vi "示波器2 - 副本 - 副本.vi"() -> ()   [LabVIEW 2018]
uses:
  <instrlib>/niScope/Configure/Trigger/niScope Configure Trigger Edge.vi
  <instrlib>/niScope/Acquire/niScope Multi Read WDT.vi
panel:
  in  "Channel(s) 2":string="0" caption="触发通道"
  out "Waveform From Scope 3":waveform(dbl)(graph) caption="采集通道"
  out "Waveform From Scope 2":waveform(dbl)(graph) caption="触发"
  out "error out":errorcluster
  in  "Channel(s)":string="0" caption="采集通道"
  out "Waveform From Scope":waveform(dbl)[](graph) caption="采集通道"
  in  "Vertical Range (V)":dbl=5.0 format="%_3g"
  in  "Min. Sample Rate":dbl=10000000.0 format="%#_6p"
  in  "Min Record Length":i32=40000
  in  "Vertical Coupling":i32(ring)=1 items=["AC", "DC", "Ground"]
  in  "Trigger Slope":i32(ring) items=["Positive", "Negative"]
  in  "Coupling":u16(ring)=1 items=["AC"=0, "DC"=1, "HF Reject"=3, "LF Reject"=4, "AC Plus HF Reject"=1001]
  in  "Trigger Level (V)":dbl=0.5 caption="Trigger Level" format="%.2f"
  in  "Trigger Modifier":i32(ring)=2 items=["None"=1, "Auto Trigger"=2]
  in  "Input Impedance":u32(ring) items=["1 mega ohm"=0, "50 ohms"=2]
  in  "Resource Name":refnum<k15>="DAQ::1"
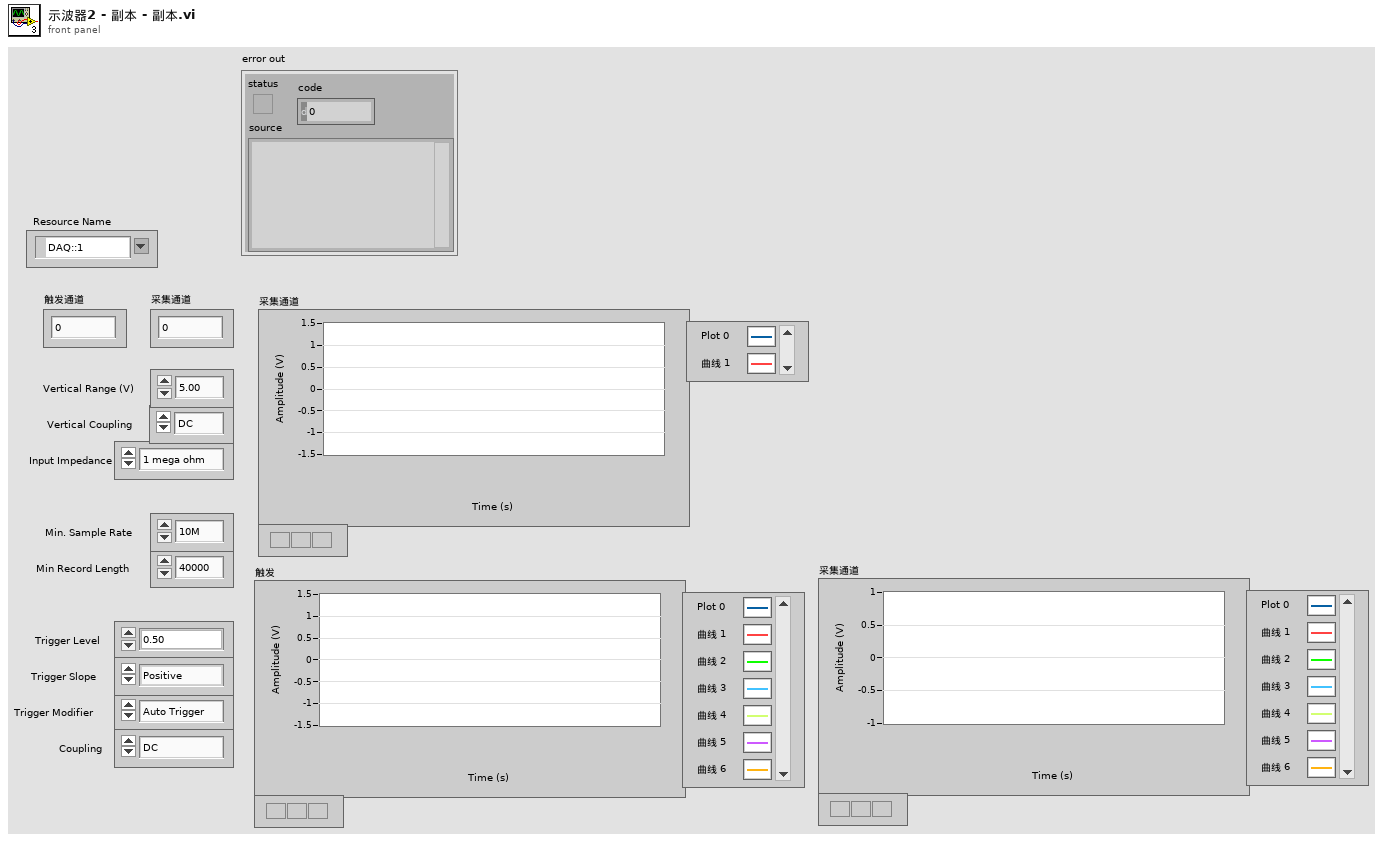
[diagram p1: front panel]
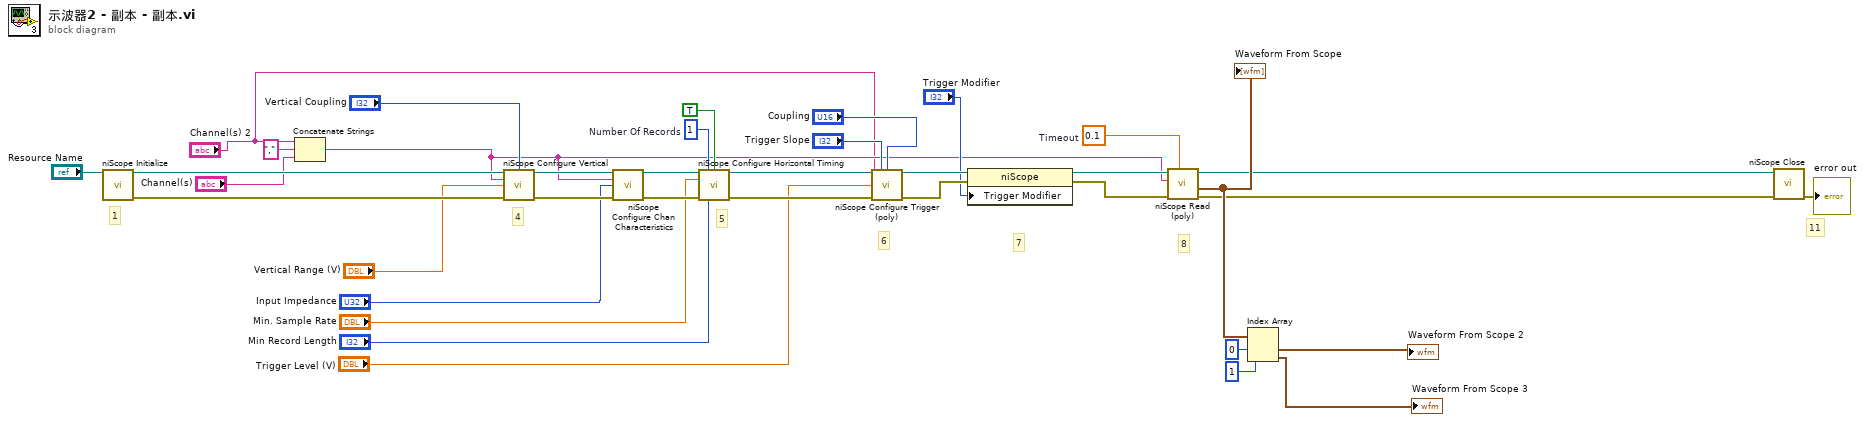
[diagram p0: block diagram]
diagram:
  w24 = 1  # Number Of Records
  w19 = 0.1  # Timeout
  # "8"
  # "6"
  # "5"
  # "4"
  # "7"
  # "11"
  # "1"
  n1 = call <instrlib>:"niScope Initialize.vi"("resource name"="Resource Name") -> ("instrument handle"=w36:refnum<k15>, "error out"=w35:errorcluster)  [unwired: 13 in]
  n2 = Concatenate Strings("Channel(s) 2", "," ("字符串"), "Channel(s)") -> (w5:string)
  n3 = call <instrlib>:"niScope Configure Vertical.vi"("instrument handle"=w36, "vertical coupling"="Vertical Coupling", "channels"=w5, "vertical range"="Vertical Range (V)", "error in"=w35) -> ("instrument handle out"=w27:refnum<k15>, "error out"=w28:errorcluster)  [unwired: 9 in]
  n4 = call <instrlib>:"niScope Configure Chan Characteristics.vi"("instrument handle"=w27, "channels"=w5, "input impedance"="Input Impedance", "error in"=w28) -> ("instrument handle out"=w26:refnum<k15>, "error out"=w25:errorcluster)  [unwired: 10 in]
  n5 = call <instrlib>:"niScope Configure Horizontal Timing.vi"("instrument handle"=w26, "number of records"=w24, "enforce realtime"=TRUE ("Enforce Realtime"), "min sample rate"="Min. Sample Rate", "error in"=w25, "min record length"="Min Record Length") -> ("instrument handle out"=w33:refnum<k15>, "error out"=w34:errorcluster)  [unwired: 8 in]
  n6 = call-poly <instrlib>:"niScope Configure Trigger (poly).vi"("instrument handle"=w33, "trigger slope"="Trigger Slope", "trigger coupling"="Coupling", "trigger source"="Channel(s) 2", "trigger level"="Trigger Level (V)", "error in"=w34) -> ("instrument handle out"=w32:refnum<k15>, "error out"=w31:errorcluster)  [unwired: 8 in]
  n7 = property class="niScope"(reference=w32, error in=w31, "Trigger Modifier"="Trigger Modifier") -> (reference out=w29:refnum<k15>, error out=w30:errorcluster)
  n8 = call-poly <instrlib>:"niScope Read (poly).vi"("timeout"=w19, "error in"=w30, "channels"=w5, "instrument handle"=w29) -> ("error out"=w2:errorcluster, "wfm"=w9:waveform(dbl)[], "instrument handle out"=w3:refnum<k15>)  [unwired: 4 in, 1 out]
  "Waveform From Scope" <- w9
  n9 = Index Array(array=w9, index #1=0 ("索引"), index #2=1 ("索引")) -> (element #1=→"Waveform From Scope 2":waveform(dbl), element #2=→"Waveform From Scope 3":waveform(dbl))
  n10 = call <instrlib>:"niScope Close.vi"("instrument handle"=w3, "error in"=w2) -> ("error out"=→"error out":errorcluster)  [unwired: 13 in]
